vi "HAL camera initialize.vi"(7 "Select camera model(s)":string[](array[string])) -> (1 "error out":errorcluster)   [LabVIEW 2016]
panel:
  in  "Quit":bool
  in  "Select Camera Number":u16(ring) items=["Camera 0", "Camera 1", "Please select a camera"]
  out "Cameras Avalable":T1(array[cluster])
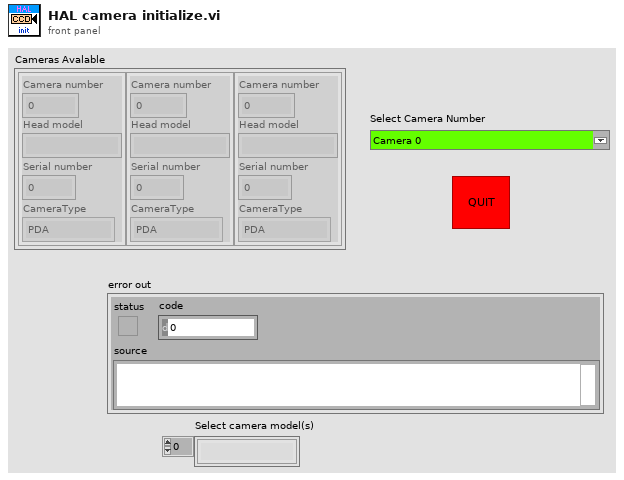
[diagram p1: front panel]
types:
  T1 = cluster{"Camera number":i32, "Head model":string, "Serial number":i32, "CameraType":enum32{"PDA", "iXon", "ICCD", "EMCCD", "CCD", "iStar", "third party camera", "iDus", "Newton", "Surcam", "USB ICCD", "Luca", "Reserved", "iKon", "InGaAs", "iVac", "Unprogrammed", "Clara", "USB iStar", "SimCam", "Neo", "iXon Ultra", "Volmos", "iVac Ultra"}}[]
  T2 = enum8{"Enabled", "Disabled", "Disabled and Grayed Out"}
  T3 = cluster{"Camera number":i32, "Head model":string, "Serial number":i32, "CameraType":enum32{"PDA", "iXon", "ICCD", "EMCCD", "CCD", "iStar", "third party camera", "iDus", "Newton", "Surcam", "USB ICCD", "Luca", "Reserved", "iKon", "InGaAs", "iVac", "Unprogrammed", "Clara", "USB iStar", "SimCam", "Neo", "iXon Ultra", "Volmos", "iVac Ultra"}}
  T4 = typedef "AndorCapabilities typedef.ctl" = cluster{"AcqModes":cluster{"single":bool, "video":bool, "accumulate":bool, "kinetic":bool, "frametransfer":bool, "fastkinetics":bool}, "ReadModes":cluster{"fullimage":bool, "subimage":bool, "singletrack":bool, "fvb":bool, "multitrack":bool, "randomtrack":bool}, "TriggerModes":cluster{"internal":bool, "external":bool}, "CameraType":enum32{"PDA", "iXon", "ICCD", "EMCCD", "CCD", "iStar", "third party camera", "iDus", "Newton", "Surcam", "USB ICCD", "Luca", "Reserved", "iKon", "InGaAs", "iVac", "Unprogrammed", "Clara", "USB iStar", "SimCam", "Neo", "iXon Ultra", "Volmos", "iVac Ultra"}, "PixelMode":cluster{"8-bit":bool, "14-bit":bool, "16-bit":bool, "32-bit":bool, "color mode":enum16{"Mono", "RGB", "CMY"}}, "SetFunctions":cluster{"vreadout":bool, "hreadout":bool, "temperature":bool, "gain":bool, "emccdgain":bool}, "GetFunctions":cluster{"temperature":bool, "targettemperature":bool, "temperaturerange":bool, "detectorsize":bool, "gain":bool, "emccdgain":bool}, "Features":cluster{"polling":bool, "events":bool, "spooling":bool, "shutter":bool}}
  T5 = enum32{"PDA", "iXon", "ICCD", "EMCCD", "CCD", "iStar", "third party camera", "iDus", "Newton", "Surcam", "USB ICCD", "Luca", "Reserved", "iKon", "InGaAs", "iVac", "Unprogrammed", "Clara", "USB iStar", "SimCam", "Neo", "iXon Ultra", "Volmos", "iVac Ultra"}
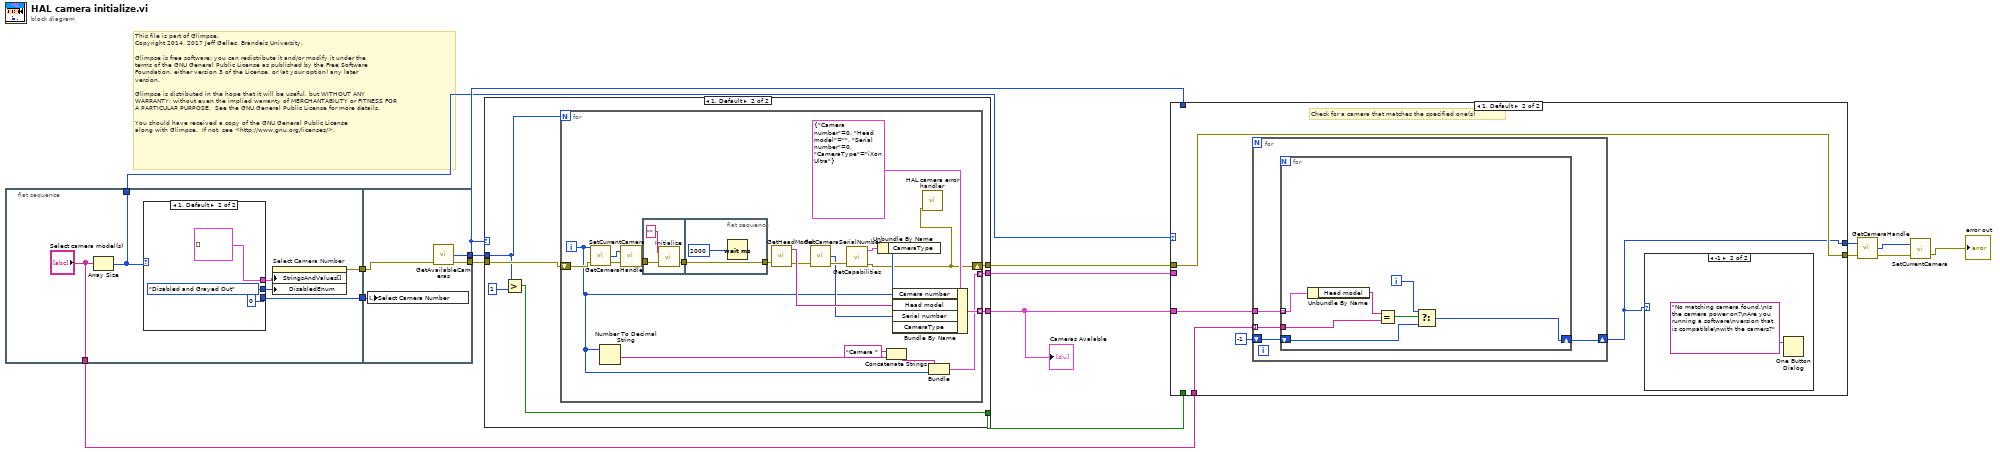
[diagram p0: block diagram]
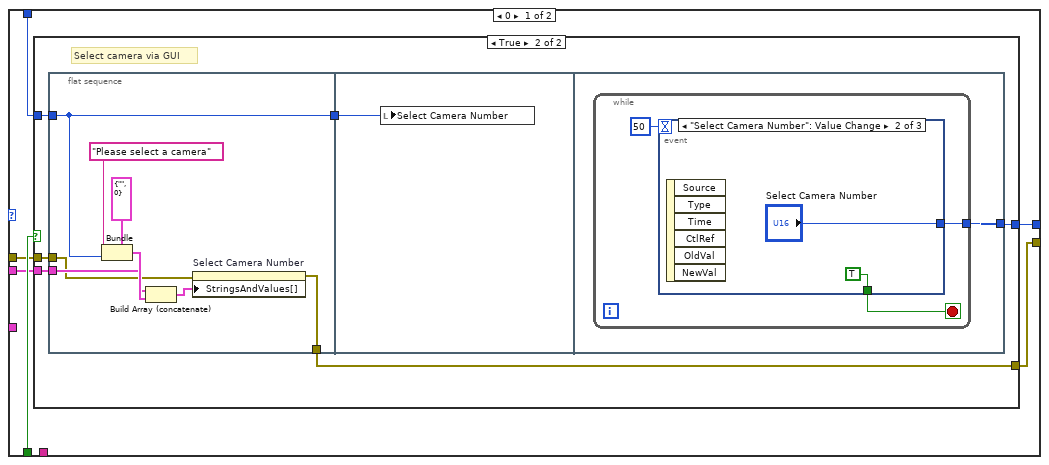
[diagram p2: hidden frame]
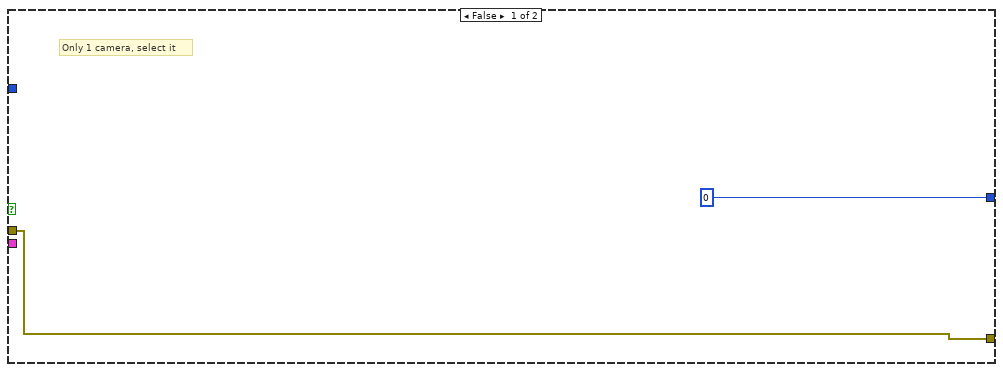
[diagram p3: hidden frame]
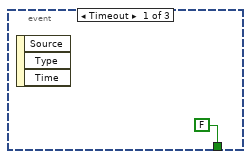
[diagram p4: hidden frame]
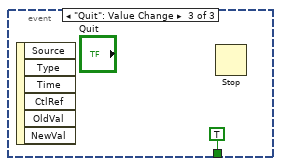
[diagram p5: hidden frame]
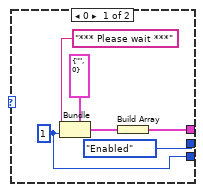
[diagram p7: hidden frame]
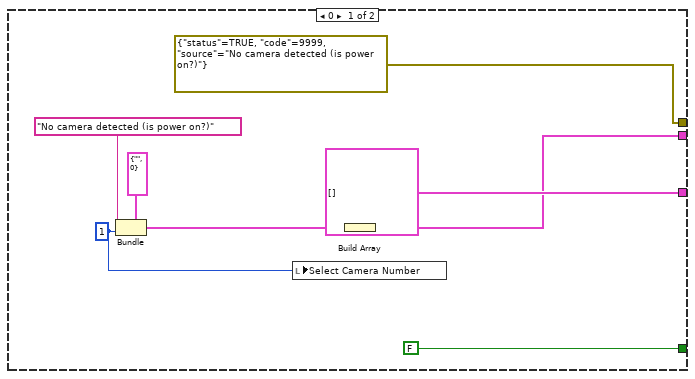
[diagram p8: hidden frame]
diagram:
  # "This file is part of Glimpse. \nCopyright 2014, 2017 Jeff Gelles, Brandeis University.    \n\nGlimpse is free software: you can redistribute it and/or modify it under the \nterms of the GNU General Public License as published by the Free Software \nFoundation, either version 3 of the License, or (at your option) any later \nversion.\n\nGlimpse is distributed in the hope that it will be useful, but WITHOUT ANY \nWARRANTY; without even the implied warranty of MERCHANTABILITY or FITNESS FOR \nA PARTICULAR PURPOSE.  See the GNU General Public License for more details.\n\nYou should have received a copy of the GNU General Public License\nalong with Glimpse.  If not, see <http://www.gnu.org/licenses/>."
  n1 = flat-sequence {
    tunnel: [w20] -> w8
    tunnel: [w19] -> w6
    tunnel: [w17] -> w3
    tunnel: ["Select camera model(s)"] -> w1
    tunnel: [w34] -> w15
    tunnel: [w33] -> w9
    tunnel: w8 -> [w31]
    tunnel: w6 -> [w32]
    frame #0 {
      n2 = Array Size(array="Select camera model(s)") -> (size(s)=w17:i32)
      n3 = case shown="1, Default" w17 {
        tunnel: [w24 cluster{string, i32}[] []] -> w21
        tunnel: [w23 0] -> w19
        tunnel: [T2."Enabled" ("Disabled") T2."Disabled and Grayed Out" ("Disabled")] -> w18
        frame 0 {
          w23 = 1
          n4 = Bundle(cluster=cluster{string, i32} {"", 0}, "*** Please wait ***", w23) -> (w25:cluster{string, i32})
          n5 = Build Array(w25) -> (w24:cluster{string, i32}[])
        }
        frame 1, Default {
        }
      }
      n6 = property on="Select Camera Number" class="Ring (strict)"("StringsAndValues[]"=w21, "DisabledEnum"=w18) -> (error out=w20:errorcluster)  [unwired: 2 in, 1 out]
    }
    frame #1 {
      n7 = local write "Select Camera Number"(w32) -> ()
      n8 = call <userlib>:"GetAvailableCameras.vi"("error in (no error)"=w31) -> ("error out"=w34:errorcluster, "totalCameras"=w33:i32)  [unwired: 2 in, 1 out]
    }
  }
  n9 = case shown="1, Default" w9 {
    tunnel: w15 -> [_ w48]
    tunnel: [T1 [] w47] -> w2
    tunnel: [errorcluster {"status"=TRUE, "code"=9999, "source"="No camera detected (is power on?)"} ("error constant") w46] -> w4
    tunnel: [FALSE w45] -> w14
    tunnel: [w37 w44] -> w5
    tunnel: w9 -> [_ w43]
    frame 0 {
      w36 = 1
      n10 = Bundle(cluster=cluster{string, i32} {"", 0}, "No camera detected (is power on?)", w36) -> (w38:cluster{string, i32})
      n11 = local write "Select Camera Number"(w36) -> ()
      n12 = Build Array(w38) -> (w37:cluster{string, i32}[])
    }
    frame 1, Default {
      n13 = Greater?(x=w43, y=1) -> (0:w45:bool)
      n14 = for {
        N: w43 -> [_]
        shift-right: [w53] -> w46
        shift-left: w48 -> [w69]
        tunnel: [w61] -> w47 mode=indexing
        tunnel: [w57] -> w44 mode=indexing
        i -> [w58]
        n15 = call <userlib>:"GetCameraHandle.vi"("error in (no error)"=w69, "cameraIndex"=w58) -> ("error out"=w68:errorcluster, "cameraHandle"=w66:i32)  [unwired: 1 in, 1 out]
        n16 = Number To Decimal String(number=w58) -> (decimal integer string=w59:string)  [unwired: 1 in]
        n17 = call <userlib>:"SetCurrentCamera.vi"("error in (no error)"=w68, "cameraHandle"=w66) -> ("error out"=w52:errorcluster)  [unwired: 1 out]
        n18 = flat-sequence {
          tunnel: w52 -> [w72]
          tunnel: [w71] -> w50
          tunnel: [w74] -> w51
          tunnel: w50 -> [w74]
          frame #0 {
            n19 = call <userlib>:"Initialize.vi"("error in (no error)"=w72, "directory (\"\")"="" ("directory (\"\")")) -> ("error out"=w71:errorcluster)  [unwired: 1 out]
          }
          frame #1 {
            n20 = Wait (ms)(milliseconds to wait=u32 2000) -> ()  [unwired: 1 out]
          }
        }
        n21 = call <userlib>:"GetHeadModel.vi"("error in (no error)"=w51) -> ("error out"=w54:errorcluster, "model"=w64:string)  [unwired: 2 in, 1 out]
        n22 = call <userlib>:"GetCameraSerialNumber.vi"("error in (no error)"=w54) -> ("error out"=w67:errorcluster, "number"=w63:i32)  [unwired: 2 in, 1 out]
        n23 = call <userlib>:"GetCapabilities.vi"("error in (no error)"=w67) -> ("error out"=w53:errorcluster, "caps"=w65:T4)  [unwired: 2 in, 1 out]
        n24 = Unbundle By Name(w65) -> ("CameraType"=w62:T5)
        n25 = Concatenate Strings("Camera " ("string"), w59) -> (w56:string)
        n26 = Bundle By Name(cluster=T3 {"Camera number"=0, "Head model"="", "Serial number"=0, "CameraType"=enum."iXon Ultra"} ("input cluster"), "Camera number"=w58, "Head model"=w64, "Serial number"=w63, "CameraType"=w62) -> (w61:T3)
        n27 = call "HAL camera error handler.vi"("error in (no error)"=w53) -> ()  [unwired: 10 in, 1 out]
        n28 = Bundle(w56, w58) -> (w57:cluster{string, i32})  [unwired: 1 in]
      }
    }
  }
  "Cameras Avalable" <- w2
  n29 = case shown="1, Default" w3 {
    tunnel: w14 -> [w80 _]
    tunnel: [w79 w106] -> w13
    tunnel: w9 -> [w78 _]
    tunnel: [w77 w108] -> w7
    tunnel: w5 -> [w76 _]
    tunnel: w4 -> [w75 w108]
    tunnel: w2 -> [_ w110]
    tunnel: w1 -> [_ w109]
    frame 0 {
      n30 = case shown="True" w80 {
        tunnel: w78 -> [_ w88]
        tunnel: [u16 0 ("Select Camera Number") w87] -> w79
        tunnel: [w81 w85] -> w77
        tunnel: w76 -> [_ w84]
        tunnel: w75 -> [w81 w83]
        frame False {
          # "Only 1 camera, select it"
        }
        frame True {
          # "Select camera via GUI"
          n31 = flat-sequence {
            tunnel: w88 -> [w93]
            tunnel: [w93] -> w86
            tunnel: [w90] -> w85
            tunnel: w84 -> [w92]
            tunnel: w83 -> [w91]
            tunnel: w86 -> [w97]
            tunnel: [w98] -> w87
            frame #0 {
              n32 = Bundle(cluster=cluster{string, i32} {"", 0}, "Please select a camera", w93) -> (w95:cluster{string, i32})
              n33 = Build Array (concatenate)(w92, w95) -> (w89:cluster{string, i32}[])
              n34 = property on="Select Camera Number" class="Ring (strict)"(error in=w91, "StringsAndValues[]"=w89) -> (error out=w90:errorcluster)  [unwired: 1 in, 1 out]
            }
            frame #1 {
              n35 = local write "Select Camera Number"(w97) -> ()
            }
            frame #2 {
              n36 = while {
                tunnel: [w99] -> w98
                stop <- w100 stop-if-true
                n37 = event shown="[1] \"Select Camera Number\": Value Change" {
                  selector: _ -> [_ _ _]
                  dyn-events: _ -> [_ _ _]
                  timeout: 50 -> [_ _ _]
                  tunnel: [FALSE TRUE TRUE] -> w100
                  tunnel: [_ "Select Camera Number" _] -> w99
                  event Timeout {
                    n38 = event-data() -> ()  [unwired: 1 in, 3 out]
                  }
                  event "Select Camera Number": Value Change {
                    n39 = event-data() -> ()  [unwired: 1 in, 6 out]
                  }
                  event "Quit": Value Change {
                    n40 = event-data() -> ()  [unwired: 1 in, 6 out]
                    n41 = Stop() -> ()  [unwired: 1 in]
                  }
                }
              }
            }
          }
        }
      }
    }
    frame 1, Default {
      # "Check for a camera that matches the specified one(s)"
      n42 = for {
        tunnel: w110 -> [w115]
        tunnel: w109 -> [w114] mode=indexing
        shift-right: [w113] -> w106
        shift-left: -1 -> [w112]
        n43 = for {
          tunnel: w115 -> [w121] mode=indexing
          tunnel: w114 -> [w122]
          shift-right: [w117] -> w113
          shift-left: w112 -> [w116]
          i -> [w118]
          n44 = Unbundle By Name(w121) -> ("Head model"=w120:string)
          n45 = Equal?(x=w120, y=w122) -> (x = y?=w119:bool)
          n46 = Select(t=w118, s=w119, f=w116) -> (s? t:f=w117:i32)
        }
      }
      n47 = case shown="-1" w106 {
        frame 0, Default {
        }
        frame -1 {
          n48 = One Button Dialog(message="No matching camera found.\nIs the camera power on?\nAre you running a software\nversion that is compatible\nwith the camers?") -> ()  [unwired: 1 in, 1 out]
        }
      }
    }
  }
  n49 = call <userlib>:"GetCameraHandle.vi"("error in (no error)"=w7, "cameraIndex"=w13) -> ("error out"=w10:errorcluster, "cameraHandle"=w12:i32)  [unwired: 1 in, 1 out]
  n50 = call <userlib>:"SetCurrentCamera.vi"("error in (no error)"=w10, "cameraHandle"=w12) -> ("error out"=→"error out":errorcluster)  [unwired: 1 out]
